vi "Find FPGA Addons.vi"(8 "error in":errorcluster, 11 "target in":refnum<k24>) -> (0 "error out":errorcluster, 1 "found ?":bool, 2 "FPGA addon refnums out":T1[](array[typedef]) format="%.0x", 3 "target out":refnum<k24>)   [LabVIEW 2021, in "Scripting API.lvlib"]
doc: "Searches the specified system definition target for FPGA addon custom devices. If found, this VI will return an array of custom device references."
uses:
  Scripting API.lvlib
  NationalInstruments.VeriStand.SystemDefinitionAPI
  <vilib>/NI VeriStand/Custom Device API/Custom Device Item Ref.ctl
  Addon/Addon Shared/SubVIs/Constants.vi
  <vilib>/NI VeriStand/Custom Device API/Custom Device API.lvlib
  Addon/Addon Shared/FPGA Addon Shared.lvlib
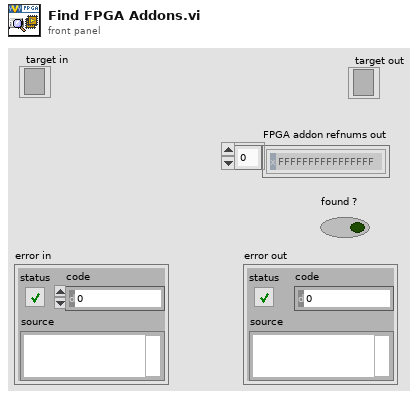
[diagram p1: front panel]
types:
  T1 = typedef "Custom Device API.lvlib/Custom Device Item Ref.ctl" = u64
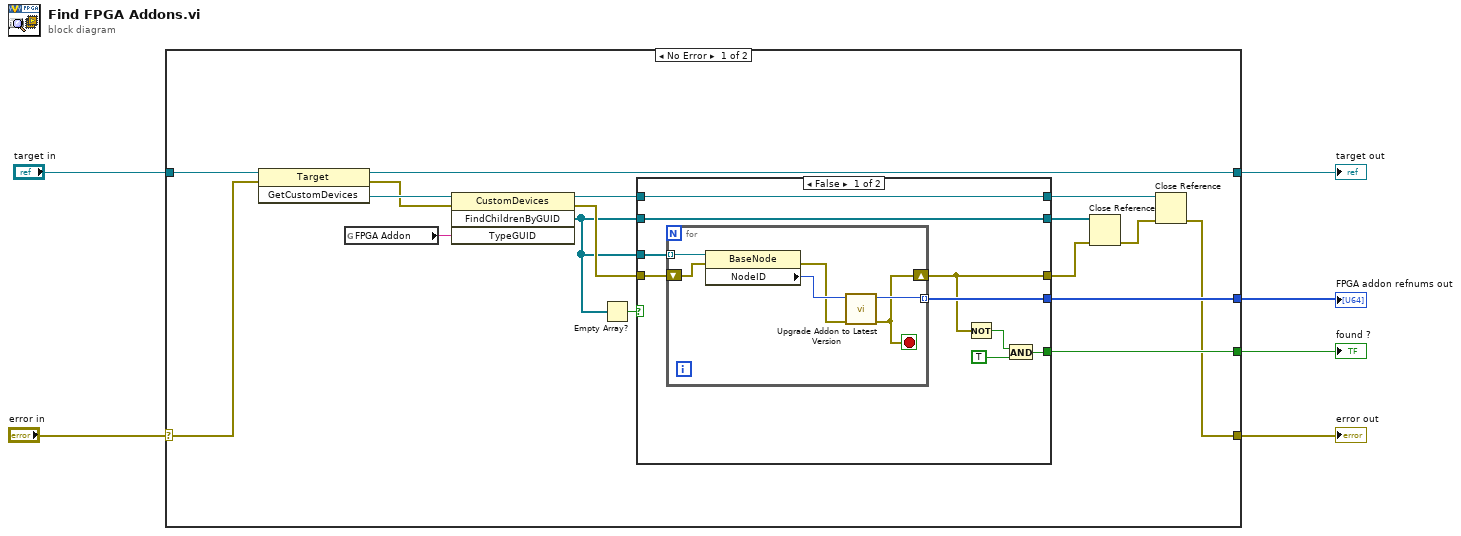
[diagram p0: block diagram]
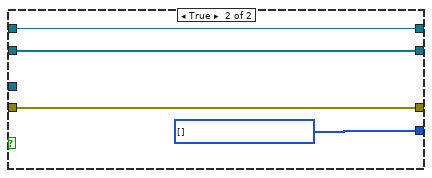
[diagram p2: hidden frame]
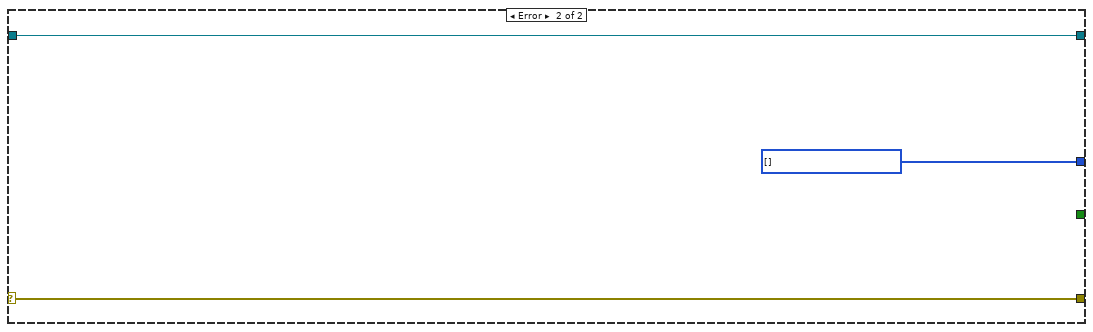
[diagram p3: hidden frame]
diagram:
  n1 = case shown="No Error" "error in" {
    selector: "error in" -> [w21 w45]
    tunnel: [w23 w43] -> w6
    tunnel: [w7 w45] -> w2
    tunnel: [w18 _] -> w5
    tunnel: [w14 T1[] []] -> w1
    tunnel: "target in" -> [w13 w43]
    frame No Error {
      n2 = invoke class="Target" method="GetCustomDevices"(reference=w13, error in=w21) -> (reference out=w23:refnum<k24>, error out=w20:errorcluster, "GetCustomDevices"=w22:refnum<k24>)  [unwired: 1 in]
      n3 = global read "Constants.vi" "FPGA Addon"() -> (w16:string)
      n4 = invoke class="CustomDevices" method="FindChildrenByGUID"(reference=w22, error in=w20, "TypeGUID"=w16) -> (reference out=w17:refnum<k24>, error out=w19:errorcluster, "FindChildrenByGUID"=w12:refnum<k24>[])  [unwired: 1 in, 1 out]
      n5 = Empty Array?(array=w12) -> (empty?=w15:bool)
      n6 = case shown="False" w15 {
        tunnel: w19 -> [w32 w42]
        tunnel: [w25 w42] -> w11
        tunnel: [w24 _] -> w18
        tunnel: w17 -> [w28 w41]
        tunnel: w12 -> [w31 _]
        tunnel: [w30 T1[] []] -> w14
        tunnel: w12 -> [w29 w40]
        tunnel: [w29 w40] -> w10
        tunnel: [w28 w41] -> w9
        frame False {
          n7 = for {
            shift-right: [w33] -> w25
            shift-left: w32 -> [w38]
            tunnel: w31 -> [w37] mode=indexing
            tunnel: [w35] -> w30 mode=indexing
            stop <- w33 stop-if-true
            n8 = property class="BaseNode"(reference=w37, error in=w38) -> (error out=w34:errorcluster, "NodeID"=w36:u64)  [unwired: 1 out]
            n9 = call "Upgrade Addon to Latest Version.vi"("error in (no error)"=w34, "Device Item Ref in in"=w36) -> ("error out"=w33:errorcluster, "Device Item Ref out"=w35:T1)  [unwired: 8 in]
          }
          n10 = Not(x=w25) -> (.not. x?=w26:bool)
          n11 = And(x=w26, y=TRUE) -> (x .and. y?=w24:bool)
        }
        frame True {
        }
      }
      n12 = Close Reference(reference=w10, error in (no error)=w11) -> (error out=w8:errorcluster)
      n13 = Close Reference(reference=w9, error in (no error)=w8) -> (error out=w7:errorcluster)
    }
    frame Error {
    }
  }
  "target out" <- w6
  "error out" <- w2
  "found ?" <- w5
  "FPGA addon refnums out" <- w1
